vi "g2Cal 80 MHz host.vi"() -> ()   [LabVIEW 2015]
uses:
  <vilib>/rvi/interface/nirviOpenFPGA/nirviOpenFPGA.xnode
  <vilib>/rvi/interface/nirviMethod/nirviMethod.xnode
  <vilib>/FPGAPlugInAG/Dynamic/niLvFpga_ReadFifo_Dynamic.vi
  <vilib>/rvi/errors/niLvFpgaMergeErrorWithErrorCode.vi
  <vilib>/rvi/interface/nirviReadWriteControl/nirviReadWriteControl.xnode
  FPGA Bitfiles/labviewintegrati_FPGATarget_g2Calsimulation2_d2xvEvYO7jw.lvbitx
  g2Cal simulation.vi
  <vilib>/FPGAPlugInAG/USB-7845R/niLvFpga_Open_USB-7845R.vi
  <vilib>/rvi/interface/common/dynamic/niFpgaDynamicAddResources.vi
  NiFpgaLv.dll
  <vilib>/Utility/error.llb/Error Cluster From Error Code.vi
  <vilib>/rvi/interface/Simulation/niFpgaSimulationCallBeginRW.vi
  <vilib>/rvi/errors/niLvFpgaAdjustHostInterfaceError.vi
panel:
  in  "Random":bool
  in  "Frequency (MHz)":fxp<+,32,4>=1.0
  out "웨이브폼 그래프":u32[](graph)
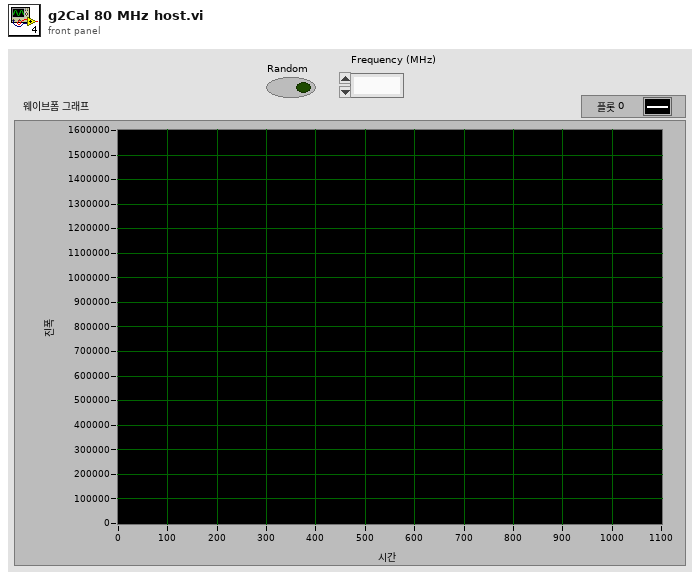
[diagram p1: front panel]
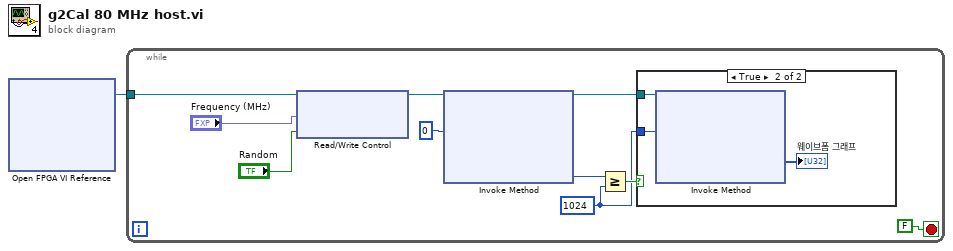
[diagram p0: block diagram]
diagram:
  n1 = xnode "Open FPGA VI Reference"() -> ("FPGA VI Reference Out"=w1:refnum<k20>)  [unwired: 2 in, 1 out]
  n2 = while {
    tunnel: w1 -> [w6]
    stop <- FALSE stop-if-true
    w3 = u32 1024 ("y")
    n3 = xnode "Read/Write Control"("FPGA VI Reference In"=w6, "Frequency (MHz)"="Frequency (MHz)", "Random"="Random") -> ("FPGA VI Reference Out"=w5:refnum<k20>)  [unwired: 1 in, 1 out]
    n4 = xnode "Invoke Method"("FPGA VI Reference In"=w5, "Number of Elements"=u32 0 ("원소의 개수")) -> ("FPGA VI Reference Out"=w8:refnum<k20>, "Elements Remaining"=w10:u32)  [unwired: 2 in, 2 out]
    n5 = Greater Or Equal?(x=w10, y=w3) -> (x >= y?=w9:bool)
    n6 = case shown="True" w9 {
      tunnel: w8 -> [_ w14]
      tunnel: w3 -> [_ w12]
      frame False {
      }
      frame True {
        n7 = xnode "Invoke Method"("FPGA VI Reference In"=w14, "Number of Elements"=w12) -> ("Data"=→"웨이브폼 그래프":u32[])  [unwired: 2 in, 3 out]
      }
    }
  }
